vi "RTS Door Delay.vi"(4 "Relay Number":u8=1 min=1 max=3 step=1, 6 "Station #":u8=1 min=1 max=8 step=1, 8 "Error In":errorcluster, 11 "Door Opening Controller Input":T1 {"Chamber 1-1"."Start Time" format="%<%X\n%x>T"; "Chamber 1-1"."End Time" format="%<%X\n%x>T"; "Time Count (s)" format="%.2f"}) -> (0 "Error Out":errorcluster, 3 "Door Opening Controller Output":T1 {"Chamber 1-1"."Start Time" format="%<%X\n%x>T"; "Chamber 1-1"."End Time" format="%<%X\n%x>T"; "Time Count (s)" format="%.2f"})   [LabVIEW 2016]
uses:
  Type Definitions/RTS Door Opener Indicator.ctl
  Type Definitions/RTS Door Ops Client.ctl
  Type Definitions/RTS Door Opening Schedule.ctl
  Type Definitions/RTS Door Ops Sequence.ctl
panel:
  out "8-3":dbl format="%.2f"
  out "8-2":dbl format="%.2f"
  out "8-1":dbl format="%.2f"
  out "7-3":dbl format="%.2f"
  out "7-2":dbl format="%.2f"
  out "7-1":dbl format="%.2f"
  out "6-3":dbl format="%.2f"
  out "6-2":dbl format="%.2f"
  out "6-1":dbl format="%.2f"
  out "5-3":dbl format="%.2f"
  out "5-2":dbl format="%.2f"
  out "5-1":dbl format="%.2f"
  out "4-3":dbl format="%.2f"
  out "4-2":dbl format="%.2f"
  out "4-1":dbl format="%.2f"
  out "3-3":dbl format="%.2f"
  out "3-2":dbl format="%.2f"
  out "3-1":dbl format="%.2f"
  out "2-3":dbl format="%.2f"
  out "2-2":dbl format="%.2f"
  out "2-1":dbl format="%.2f"
  out "1-3":dbl format="%.2f"
  out "1-2":dbl format="%.2f"
  out "1-1":dbl format="%.2f"
  # "Individual Timers"
  # "Chamber Conditions:"
  # "Chamber Conditions:"
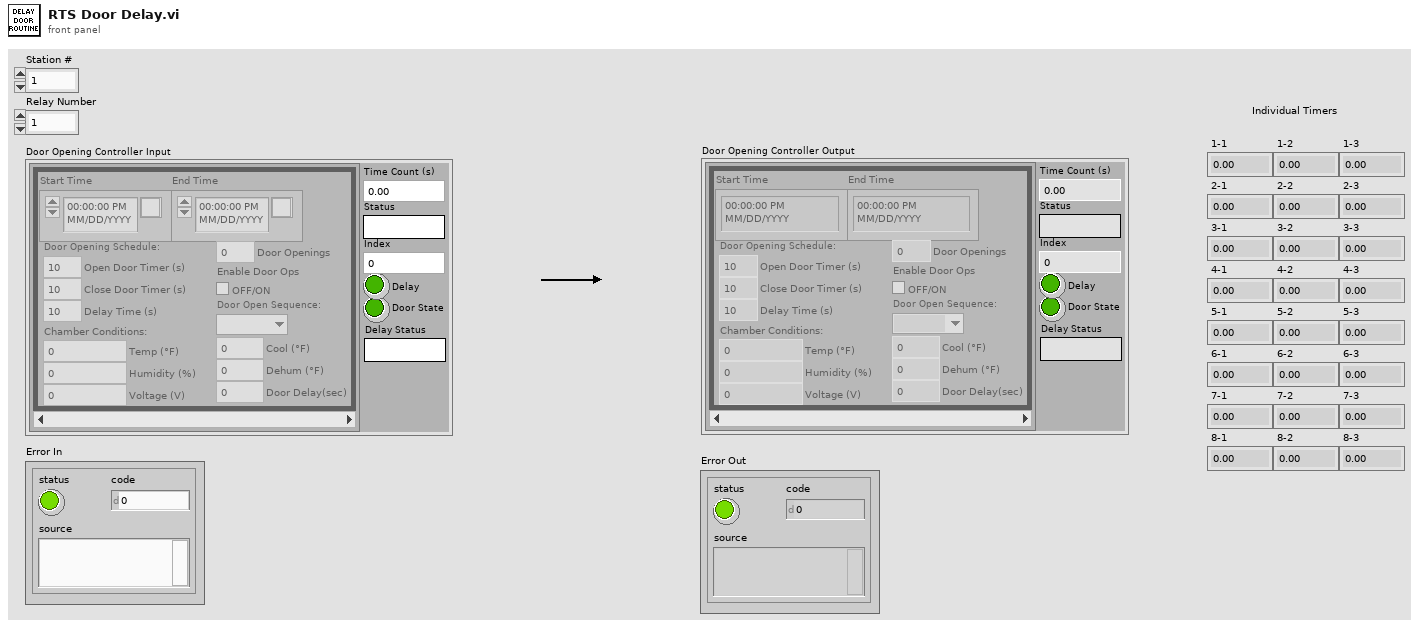
[diagram p1: front panel]
types:
  T1 = typedef "RTS Door Opener Indicator.ctl" = cluster{"Time Count (s)":dbl, "Status":string, "Door State":bool, "Delay":bool, "Chamber 1-1":T2[], "Index":i32, "Delay Status":string}
  T2 = typedef "RTS Door Ops Client.ctl" = cluster{"End Time":timestamp, "Start Time":timestamp, "Door Opening Schedule:":T3, "Enable Door Ops":bool, "Door Openings":u32, "Temp (°F)":dbl, "Humidity (%)":dbl, "Voltage (V)":dbl, "Door Open Sequence:":T4, "Door Delay(sec)":dbl, "Dehum (°F)":dbl, "Cool (°F)":dbl}
  T3 = typedef "RTS Door Opening Schedule.ctl" = cluster{"Open Door Timer (s)":dbl, "Delay Time (s)":dbl, "Close Door Timer (s)":dbl}
  T4 = typedef "RTS Door Ops Sequence.ctl" = enum16{"", "1st", "2nd", "3rd"}
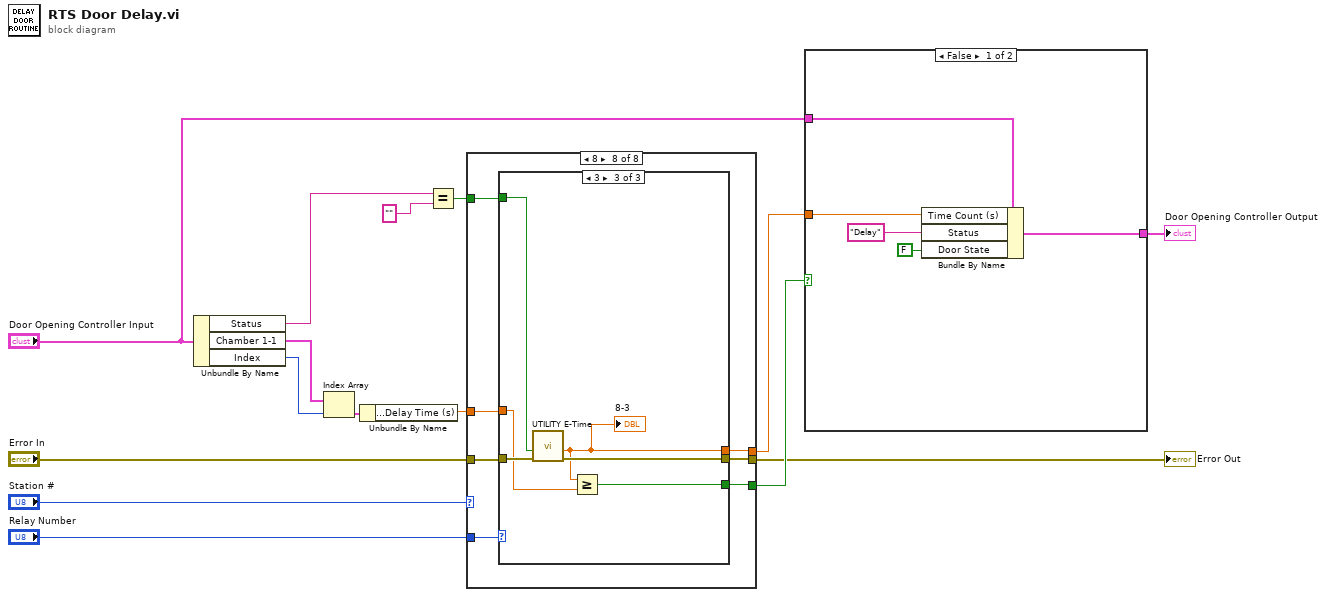
[diagram p0: block diagram]
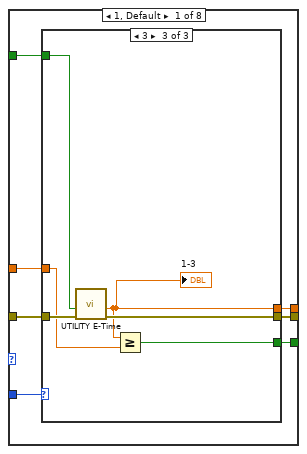
[diagram p2: hidden frame]
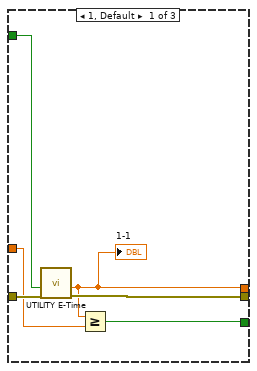
[diagram p3: hidden frame]
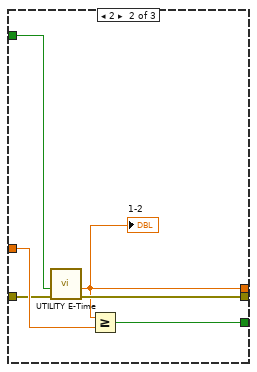
[diagram p4: hidden frame]
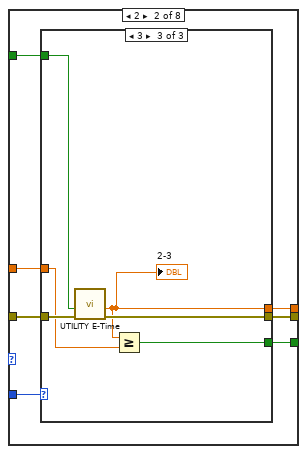
[diagram p5: hidden frame]
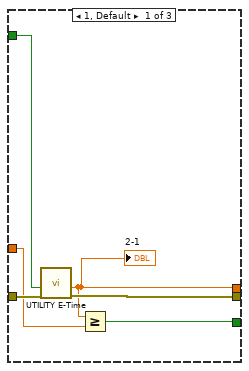
[diagram p6: hidden frame]
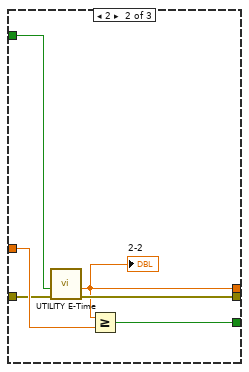
[diagram p7: hidden frame]
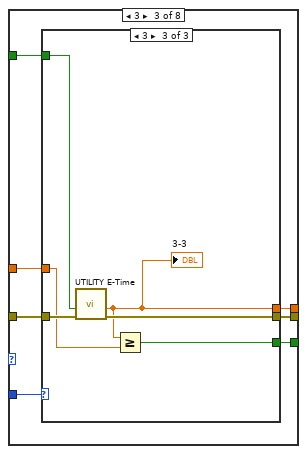
[diagram p8: hidden frame]
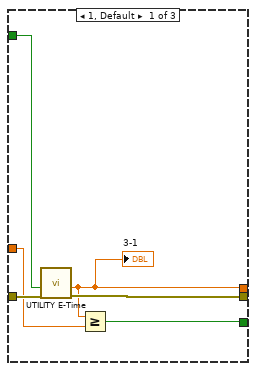
[diagram p9: hidden frame]
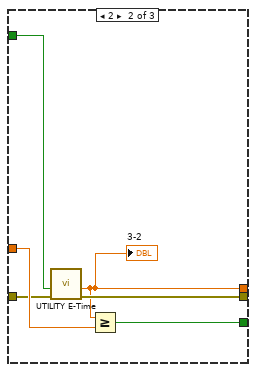
[diagram p10: hidden frame]
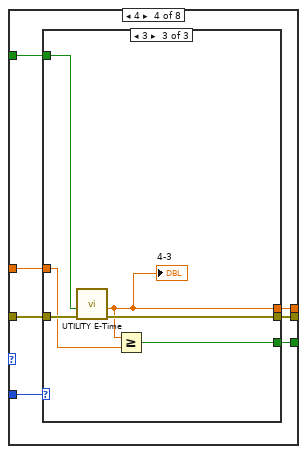
[diagram p11: hidden frame]
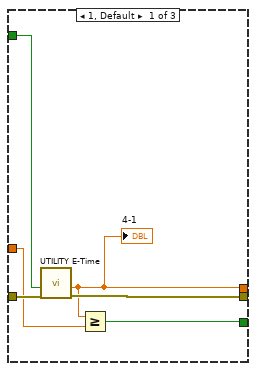
[diagram p12: hidden frame]
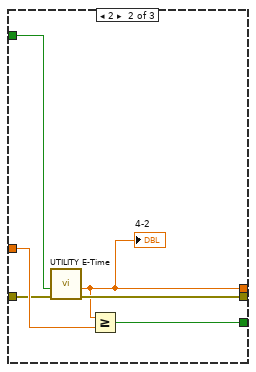
[diagram p13: hidden frame]
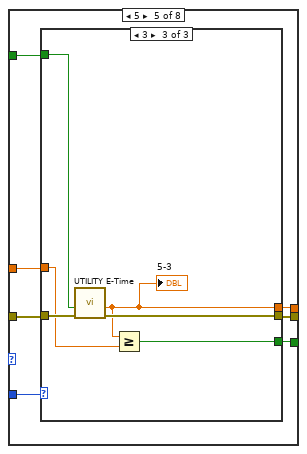
[diagram p14: hidden frame]
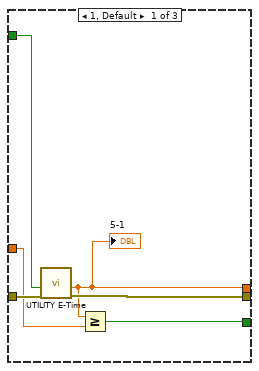
[diagram p15: hidden frame]
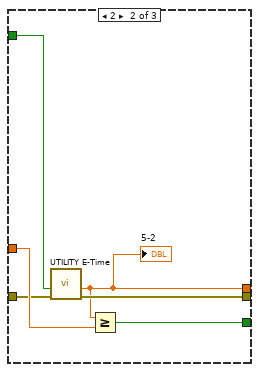
[diagram p16: hidden frame]
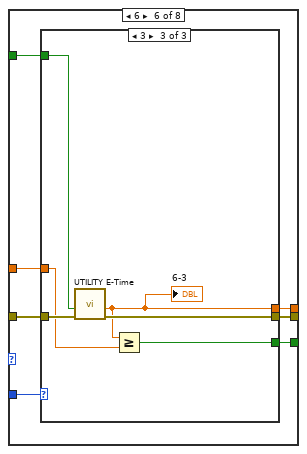
[diagram p17: hidden frame]
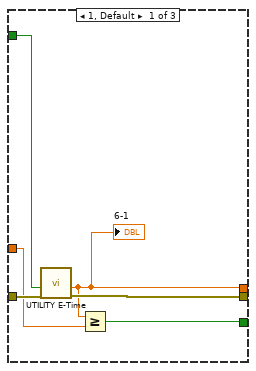
[diagram p18: hidden frame]
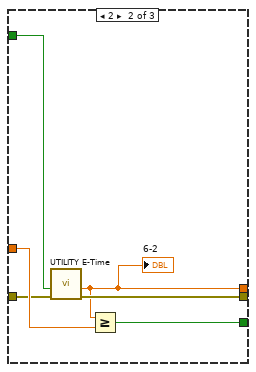
[diagram p19: hidden frame]
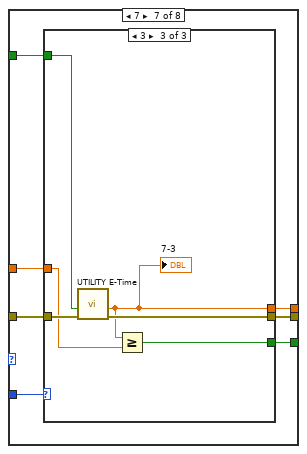
[diagram p20: hidden frame]
diagram:
  n1 = Unbundle By Name("Door Opening Controller Input") -> ("Status"=w13:string, "Chamber 1-1"=w11:T2[], "Index"=w10:i32)
  n2 = Index Array(array=w11, index=w10) -> (element=w9:T2)
  n3 = Unbundle By Name(w9) -> ("Door Opening Schedule:.Delay Time (s)"=w8:dbl)
  n4 = Equal?(x=w13, y="") -> (x = y?=w5:bool)
  n5 = case shown="8" "Station #" {
    tunnel: [w22 w43 w68 w93 w118 w143 w168 w193] -> w4
    tunnel: [w21 w42 w67 w91 w116 w141 w167 w191] -> w3
    tunnel: [w20 w44 w69 w92 w117 w142 w169 w192] -> w1
    tunnel: "Error In" -> [w19 w45 w70 w95 w120 w145 w170 w195]
    tunnel: w5 -> [w18 w46 w72 w97 w122 w147 w172 w197]
    tunnel: w8 -> [w17 w41 w71 w96 w121 w146 w171 w196]
    tunnel: "Relay Number" -> [w16 w47 w66 w94 w119 w144 w166 w194]
    frame 1, Default {
      n6 = case shown="3" w16 {
        tunnel: [w26 w29 w35] -> w22
        tunnel: [w25 w32 w38] -> w21
        tunnel: [w27 w30 w39] -> w20
        tunnel: w19 -> [w28 w31 w40]
        tunnel: w18 -> [w23 w34 w36]
        tunnel: w17 -> [w24 w33 w37]
        frame 1, Default {
          n7 = call "UTILITY E-Time.vi"("error in (no error)"=w28, "Reset"=w23) -> ("error out"=w27:errorcluster, "Elapsed Time (sec)"=w26:dbl)  [unwired: 7 in, 1 out]
          "1-1" <- w26
          n8 = Greater Or Equal?(x=w26, y=w24) -> (x >= y?=w25:bool)
        }
        frame 2 {
          n9 = call "UTILITY E-Time.vi"("error in (no error)"=w31, "Reset"=w34) -> ("error out"=w30:errorcluster, "Elapsed Time (sec)"=w29:dbl)  [unwired: 7 in, 1 out]
          "1-2" <- w29
          n10 = Greater Or Equal?(x=w29, y=w33) -> (x >= y?=w32:bool)
        }
        frame 3 {
          n11 = call "UTILITY E-Time.vi"("error in (no error)"=w40, "Reset"=w36) -> ("error out"=w39:errorcluster, "Elapsed Time (sec)"=w35:dbl)  [unwired: 7 in, 1 out]
          "1-3" <- w35
          n12 = Greater Or Equal?(x=w35, y=w37) -> (x >= y?=w38:bool)
        }
      }
    }
    frame 2 {
      n13 = case shown="3" w47 {
        tunnel: [w48 w54 w60] -> w43
        tunnel: [w51 w57 w63] -> w42
        tunnel: [w52 w55 w64] -> w44
        tunnel: w45 -> [w53 w56 w65]
        tunnel: w46 -> [w49 w59 w61]
        tunnel: w41 -> [w50 w58 w62]
        frame 1, Default {
          n14 = call "UTILITY E-Time.vi"("error in (no error)"=w53, "Reset"=w49) -> ("error out"=w52:errorcluster, "Elapsed Time (sec)"=w48:dbl)  [unwired: 7 in, 1 out]
          "2-1" <- w48
          n15 = Greater Or Equal?(x=w48, y=w50) -> (x >= y?=w51:bool)
        }
        frame 2 {
          n16 = call "UTILITY E-Time.vi"("error in (no error)"=w56, "Reset"=w59) -> ("error out"=w55:errorcluster, "Elapsed Time (sec)"=w54:dbl)  [unwired: 7 in, 1 out]
          "2-2" <- w54
          n17 = Greater Or Equal?(x=w54, y=w58) -> (x >= y?=w57:bool)
        }
        frame 3 {
          n18 = call "UTILITY E-Time.vi"("error in (no error)"=w65, "Reset"=w61) -> ("error out"=w64:errorcluster, "Elapsed Time (sec)"=w60:dbl)  [unwired: 7 in, 1 out]
          "2-3" <- w60
          n19 = Greater Or Equal?(x=w60, y=w62) -> (x >= y?=w63:bool)
        }
      }
    }
    frame 3 {
      n20 = case shown="3" w66 {
        tunnel: [w73 w79 w85] -> w68
        tunnel: [w76 w82 w88] -> w67
        tunnel: [w77 w80 w89] -> w69
        tunnel: w70 -> [w78 w81 w90]
        tunnel: w72 -> [w74 w84 w86]
        tunnel: w71 -> [w75 w83 w87]
        frame 1, Default {
          n21 = call "UTILITY E-Time.vi"("error in (no error)"=w78, "Reset"=w74) -> ("error out"=w77:errorcluster, "Elapsed Time (sec)"=w73:dbl)  [unwired: 7 in, 1 out]
          "3-1" <- w73
          n22 = Greater Or Equal?(x=w73, y=w75) -> (x >= y?=w76:bool)
        }
        frame 2 {
          n23 = call "UTILITY E-Time.vi"("error in (no error)"=w81, "Reset"=w84) -> ("error out"=w80:errorcluster, "Elapsed Time (sec)"=w79:dbl)  [unwired: 7 in, 1 out]
          "3-2" <- w79
          n24 = Greater Or Equal?(x=w79, y=w83) -> (x >= y?=w82:bool)
        }
        frame 3 {
          n25 = call "UTILITY E-Time.vi"("error in (no error)"=w90, "Reset"=w86) -> ("error out"=w89:errorcluster, "Elapsed Time (sec)"=w85:dbl)  [unwired: 7 in, 1 out]
          "3-3" <- w85
          n26 = Greater Or Equal?(x=w85, y=w87) -> (x >= y?=w88:bool)
        }
      }
    }
    frame 4 {
      n27 = case shown="3" w94 {
        tunnel: [w98 w104 w110] -> w93
        tunnel: [w101 w107 w113] -> w91
        tunnel: [w102 w105 w114] -> w92
        tunnel: w95 -> [w103 w106 w115]
        tunnel: w97 -> [w99 w109 w111]
        tunnel: w96 -> [w100 w108 w112]
        frame 1, Default {
          n28 = call "UTILITY E-Time.vi"("error in (no error)"=w103, "Reset"=w99) -> ("error out"=w102:errorcluster, "Elapsed Time (sec)"=w98:dbl)  [unwired: 7 in, 1 out]
          "4-1" <- w98
          n29 = Greater Or Equal?(x=w98, y=w100) -> (x >= y?=w101:bool)
        }
        frame 2 {
          n30 = call "UTILITY E-Time.vi"("error in (no error)"=w106, "Reset"=w109) -> ("error out"=w105:errorcluster, "Elapsed Time (sec)"=w104:dbl)  [unwired: 7 in, 1 out]
          "4-2" <- w104
          n31 = Greater Or Equal?(x=w104, y=w108) -> (x >= y?=w107:bool)
        }
        frame 3 {
          n32 = call "UTILITY E-Time.vi"("error in (no error)"=w115, "Reset"=w111) -> ("error out"=w114:errorcluster, "Elapsed Time (sec)"=w110:dbl)  [unwired: 7 in, 1 out]
          "4-3" <- w110
          n33 = Greater Or Equal?(x=w110, y=w112) -> (x >= y?=w113:bool)
        }
      }
    }
    frame 5 {
      n34 = case shown="3" w119 {
        tunnel: [w123 w129 w135] -> w118
        tunnel: [w126 w132 w138] -> w116
        tunnel: [w127 w130 w139] -> w117
        tunnel: w120 -> [w128 w131 w140]
        tunnel: w122 -> [w124 w134 w136]
        tunnel: w121 -> [w125 w133 w137]
        frame 1, Default {
          n35 = call "UTILITY E-Time.vi"("error in (no error)"=w128, "Reset"=w124) -> ("error out"=w127:errorcluster, "Elapsed Time (sec)"=w123:dbl)  [unwired: 7 in, 1 out]
          "5-1" <- w123
          n36 = Greater Or Equal?(x=w123, y=w125) -> (x >= y?=w126:bool)
        }
        frame 2 {
          n37 = call "UTILITY E-Time.vi"("error in (no error)"=w131, "Reset"=w134) -> ("error out"=w130:errorcluster, "Elapsed Time (sec)"=w129:dbl)  [unwired: 7 in, 1 out]
          "5-2" <- w129
          n38 = Greater Or Equal?(x=w129, y=w133) -> (x >= y?=w132:bool)
        }
        frame 3 {
          n39 = call "UTILITY E-Time.vi"("error in (no error)"=w140, "Reset"=w136) -> ("error out"=w139:errorcluster, "Elapsed Time (sec)"=w135:dbl)  [unwired: 7 in, 1 out]
          "5-3" <- w135
          n40 = Greater Or Equal?(x=w135, y=w137) -> (x >= y?=w138:bool)
        }
      }
    }
    frame 6 {
      n41 = case shown="3" w144 {
        tunnel: [w148 w154 w160] -> w143
        tunnel: [w151 w157 w163] -> w141
        tunnel: [w152 w155 w164] -> w142
        tunnel: w145 -> [w153 w156 w165]
        tunnel: w147 -> [w149 w159 w161]
        tunnel: w146 -> [w150 w158 w162]
        frame 1, Default {
          n42 = call "UTILITY E-Time.vi"("error in (no error)"=w153, "Reset"=w149) -> ("error out"=w152:errorcluster, "Elapsed Time (sec)"=w148:dbl)  [unwired: 7 in, 1 out]
          "6-1" <- w148
          n43 = Greater Or Equal?(x=w148, y=w150) -> (x >= y?=w151:bool)
        }
        frame 2 {
          n44 = call "UTILITY E-Time.vi"("error in (no error)"=w156, "Reset"=w159) -> ("error out"=w155:errorcluster, "Elapsed Time (sec)"=w154:dbl)  [unwired: 7 in, 1 out]
          "6-2" <- w154
          n45 = Greater Or Equal?(x=w154, y=w158) -> (x >= y?=w157:bool)
        }
        frame 3 {
          n46 = call "UTILITY E-Time.vi"("error in (no error)"=w165, "Reset"=w161) -> ("error out"=w164:errorcluster, "Elapsed Time (sec)"=w160:dbl)  [unwired: 7 in, 1 out]
          "6-3" <- w160
          n47 = Greater Or Equal?(x=w160, y=w162) -> (x >= y?=w163:bool)
        }
      }
    }
    frame 7 {
      n48 = case shown="3" w166 {
        tunnel: [w173 w179 w185] -> w168
        tunnel: [w176 w182 w188] -> w167
        tunnel: [w177 w180 w189] -> w169
        tunnel: w170 -> [w178 w181 w190]
        tunnel: w172 -> [w174 w184 w186]
        tunnel: w171 -> [w175 w183 w187]
        frame 1, Default {
          n49 = call "UTILITY E-Time.vi"("error in (no error)"=w178, "Reset"=w174) -> ("error out"=w177:errorcluster, "Elapsed Time (sec)"=w173:dbl)  [unwired: 7 in, 1 out]
          "7-1" <- w173
          n50 = Greater Or Equal?(x=w173, y=w175) -> (x >= y?=w176:bool)
        }
        frame 2 {
          n51 = call "UTILITY E-Time.vi"("error in (no error)"=w181, "Reset"=w184) -> ("error out"=w180:errorcluster, "Elapsed Time (sec)"=w179:dbl)  [unwired: 7 in, 1 out]
          "7-2" <- w179
          n52 = Greater Or Equal?(x=w179, y=w183) -> (x >= y?=w182:bool)
        }
        frame 3 {
          n53 = call "UTILITY E-Time.vi"("error in (no error)"=w190, "Reset"=w186) -> ("error out"=w189:errorcluster, "Elapsed Time (sec)"=w185:dbl)  [unwired: 7 in, 1 out]
          "7-3" <- w185
          n54 = Greater Or Equal?(x=w185, y=w187) -> (x >= y?=w188:bool)
        }
      }
    }
    frame 8 {
      n55 = case shown="3" w194 {
        tunnel: [w198 w204 w210] -> w193
        tunnel: [w201 w207 w213] -> w191
        tunnel: [w202 w205 w214] -> w192
        tunnel: w195 -> [w203 w206 w215]
        tunnel: w197 -> [w199 w209 w211]
        tunnel: w196 -> [w200 w208 w212]
        frame 1, Default {
          n56 = call "UTILITY E-Time.vi"("error in (no error)"=w203, "Reset"=w199) -> ("error out"=w202:errorcluster, "Elapsed Time (sec)"=w198:dbl)  [unwired: 7 in, 1 out]
          "8-1" <- w198
          n57 = Greater Or Equal?(x=w198, y=w200) -> (x >= y?=w201:bool)
        }
        frame 2 {
          n58 = call "UTILITY E-Time.vi"("error in (no error)"=w206, "Reset"=w209) -> ("error out"=w205:errorcluster, "Elapsed Time (sec)"=w204:dbl)  [unwired: 7 in, 1 out]
          "8-2" <- w204
          n59 = Greater Or Equal?(x=w204, y=w208) -> (x >= y?=w207:bool)
        }
        frame 3 {
          n60 = call "UTILITY E-Time.vi"("error in (no error)"=w215, "Reset"=w211) -> ("error out"=w214:errorcluster, "Elapsed Time (sec)"=w210:dbl)  [unwired: 7 in, 1 out]
          "8-3" <- w210
          n61 = Greater Or Equal?(x=w210, y=w212) -> (x >= y?=w213:bool)
        }
      }
    }
  }
  "Error Out" <- w1
  n62 = case shown="False" w3 {
    tunnel: [w218 w223] -> w15
    tunnel: "Door Opening Controller Input" -> [w219 w222]
    tunnel: w4 -> [w217 _]
    frame False {
      n63 = Bundle By Name(cluster=w219, "Time Count (s)"=w217, "Status"="Delay" ("Boiler Status Indicators.Status"), "Door State"=FALSE ("Open Door")) -> (w218:T1)
    }
    frame True {
      n64 = Bundle By Name(cluster=w222, "Delay"=FALSE ("Pilot Indicator")) -> (w223:T1)
    }
  }
  "Door Opening Controller Output" <- w15
